vi "ROS_Master_UnregisterServiceText.vi"(1 "String w/o Tag":string) -> (0 "Cluster":T1)   [LabVIEW 2012]
doc: "Returns a cluster of service text from unregistering service with master"
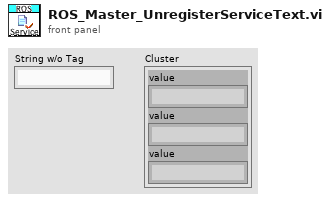
[diagram p1: front panel]
types:
  T1 = cluster{"value":string, "value":string, "value":string}
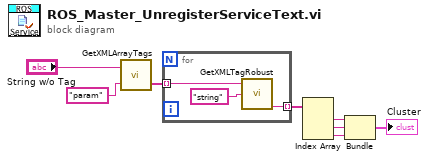
[diagram p0: block diagram]
diagram:
  n1 = call "GetXMLArrayTags.vi"("ArrayTag"="param", "String"="String w/o Tag") -> ("Array"=w6:string[])  [unwired: 1 out]
  n2 = for {
    tunnel: w6 -> [w10] mode=indexing
    tunnel: [w9] -> w7 mode=indexing
    n3 = call "GetXMLTagRobust.vi"("Tag"="string", "String"=w10) -> ("value"=w9:string)  [unwired: 1 in, 3 out]
  }
  n4 = Index Array(array=w7) -> (element #1=w2:string, element #2=w3:string, element #3=w4:string)  [unwired: 3 in]
  n5 = Bundle("value"=w2, "value"=w3, "value"=w4) -> (→"Cluster":T1)  [unwired: 1 in]
